vi "prueba_com.vi"() -> ()   [LabVIEW 2021]
uses:
  <vilib>/MakerHub/LINX/Private/Type Defs/Peripherals/I2C/EOF.ctl
  <vilib>/MakerHub/LINX/Private/Local IO/LinxI2cWrite.vi
  <vilib>/MakerHub/LINX/Public/Utilities/Check Channel.vi
  <vilib>/MakerHub/LINX/Public/Utilities/Open Serial.vi
  <vilib>/MakerHub/LINX/Private/Utilties/Generate Error.vi
  <vilib>/MakerHub/LINX/LMH-LINX.lvlib
panel:
  in  "Data":u8[](array[numeric])=[100]
  in  "EOF":T1
  out "string":string
  out "Device Name 2":string
  in  "I2C Slave Address (0)":u8=8
  out "Data 3":u8[](array[numeric])
  out "Error Out 2":errorcluster
  in  "Error In 2":errorcluster
  in  "Serial Port 2":refnum<visa-resource-name>="N/A"
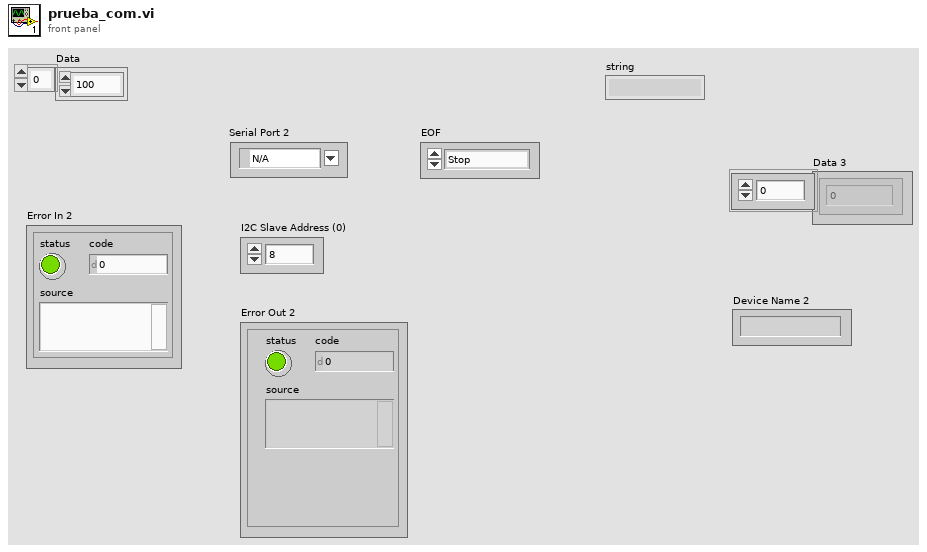
[diagram p1: front panel]
types:
  T1 = typedef "LMH-LINX.lvlib/EOF.ctl" = enum8{"Stop", "Restart", "Restart No Stop", "No Stop"}
  T2 = typedef "LMH-LINX.lvlib/LINX Ref.ctl" = cluster{"IO":T3, "Interface":T4, "LINX Device Config":T5}
  T3 = typedef "LMH-LINX.lvlib/Platform.ctl" = enum16{"Remote", "Local"}
  T4 = typedef "LMH-LINX.lvlib/Interface.ctl" = enum16{"Serial", "TCP"}
  T5 = typedef "LMH-LINX.lvlib/Device.lvlib/LINX Device Config.ctl" = cluster{"Interface":T4, "COM Port":refnum<visa-resource-name>, "TCP Configuration":T6, "Device Family":u8, "Device ID":u8, "Device Name":string, "TCP Ref":refnum<k5>, "Channels":T7}
  T6 = typedef "LMH-LINX.lvlib/Device.lvlib/TCP Config.ctl" = cluster{"IP Address":string, "Port":u16}
  T7 = typedef "LMH-LINX.lvlib/Channels.ctl" = cluster{"DI":u8[], "DO":u8[], "AI":u8[], "AO":u8[], "PWM":u8[], "QE":u8[], "UART":u8[], "I2C 2":u8[], "SPI":u8[], "CAN":u8[], "Servo":u8[], "AI Ref (V)":dbl, "AI Resolution (Bits)":u8, "AO Ref (V)":dbl, "AO Resolution (Bits)":u8}
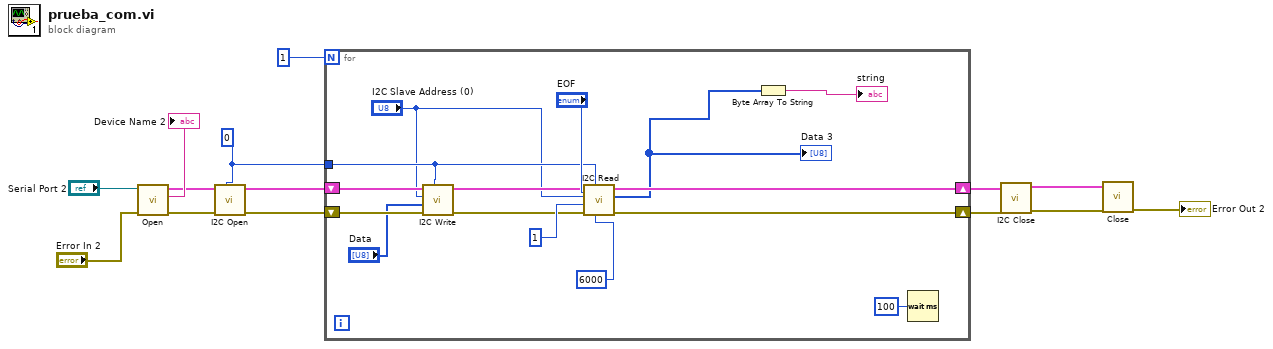
[diagram p0: block diagram]
diagram:
  w4 = u8 0 ("I2C Channel")
  n1 = call-poly <vilib>:"Open.vi"("Error In"="Error In 2", "Serial Port"="Serial Port 2") -> ("Error Out"=w10:errorcluster, "Device Name"=→"Device Name 2":string, "LINX Resource"=w3:T2)  [unwired: 7 in]
  n2 = call <vilib>:"I2C Open.vi"("I2C Channel (0)"=w4, "Error In"=w10, "LINX Resource"=w3) -> ("Error Out"=w8:errorcluster, "LINX Resource"=w6:T2)  [unwired: 7 in]
  n3 = for {
    N: 1 -> [_]
    tunnel: w4 -> [w20]
    shift-right: [w27] -> w7
    shift-left: w8 -> [w22]
    shift-right: [w26] -> w5
    shift-left: w6 -> [w19]
    n4 = call <vilib>:"I2C Write.vi"("I2C Channel"=w20, "Error In"=w22, "Data"="Data", "I2C Slave Address (0)"="I2C Slave Address (0)", "LINX Resource"=w19) -> ("Error Out"=w21:errorcluster, "LINX Resource"=w18:T2)  [unwired: 5 in]
    n5 = call <vilib>:"I2C Read.vi"("EOF"="EOF", "Timeout (1000 ms)"=u16 6000, "I2C Channel"=w20, "Error In"=w21, "Bytes To Read"=u8 1, "I2C Slave Address (0)"="I2C Slave Address (0)", "LINX Resource"=w18) -> ("Error Out"=w27:errorcluster, "Data"=w25:u8[], "LINX Resource"=w26:T2)  [unwired: 2 in]
    "Data 3" <- w25
    n6 = Byte Array To String(unsigned byte array=w25) -> (string=→"string":string)
    n7 = Wait (ms)(milliseconds to wait=u32 100) -> ()  [unwired: 1 out]
  }
  n8 = call <vilib>:"I2C Close.vi"("Error In"=w7, "LINX Resource"=w5) -> ("Error Out"=w13:errorcluster, "LINX Resource"=w12:T2)  [unwired: 8 in]
  n9 = call <vilib>:"Close.vi"("Error In"=w13, "LINX Resource"=w12) -> ("Error Out"=→"Error Out 2":errorcluster)  [unwired: 9 in]
